vi "Word_Update_Table2.vi"(0 "report in":refnum<class "NI_report.lvclass">, 5 "start":cluster{"row":i32, "column":i32}, 9 "Table Ref":refnum<k7>, 11 "error in (no error)":errorcluster, 12 "value":string[][](array[string])) -> (4 "report out":refnum<class "NI_report.lvclass">, 15 "error out":errorcluster)   [LabVIEW 2020, in "NI_Word.lvclass"]
uses:
  <vilib>/Utility/NIReport.llb/Word/NI_Word.lvclass
  <vilib>/Utility/NIReport.llb/NI_report.lvclass
  C:/Program Files (x86)/National Instruments/LabVIEW 2020/vi.lib/Utility/NIReport.llb/NI_report.lvclass
  <vilib>/Utility/NIReport.llb/Word/NI_Word.lvclass/NI_Word.ctl
  <vilib>/Utility/NIReport.llb/NI_ReportGenerationCore.lvlib
panel:
  # "This is a copy of the Word_Update_Table.vi specifically used by\nthe MS Office Report Express VI to update the contents of\na table where the bookmark consists of a group of table cells."
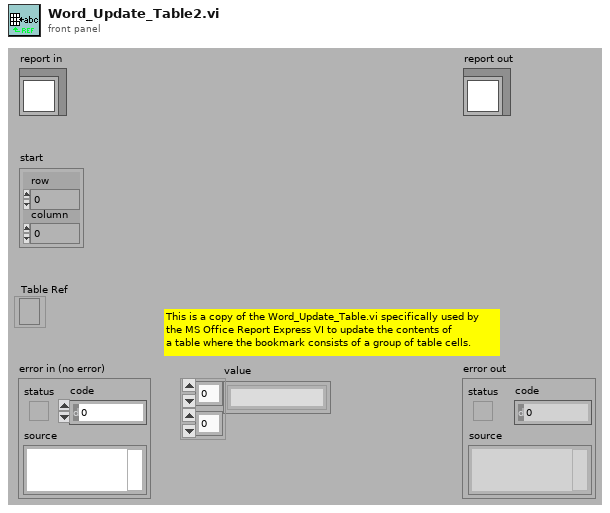
[diagram p1: front panel]
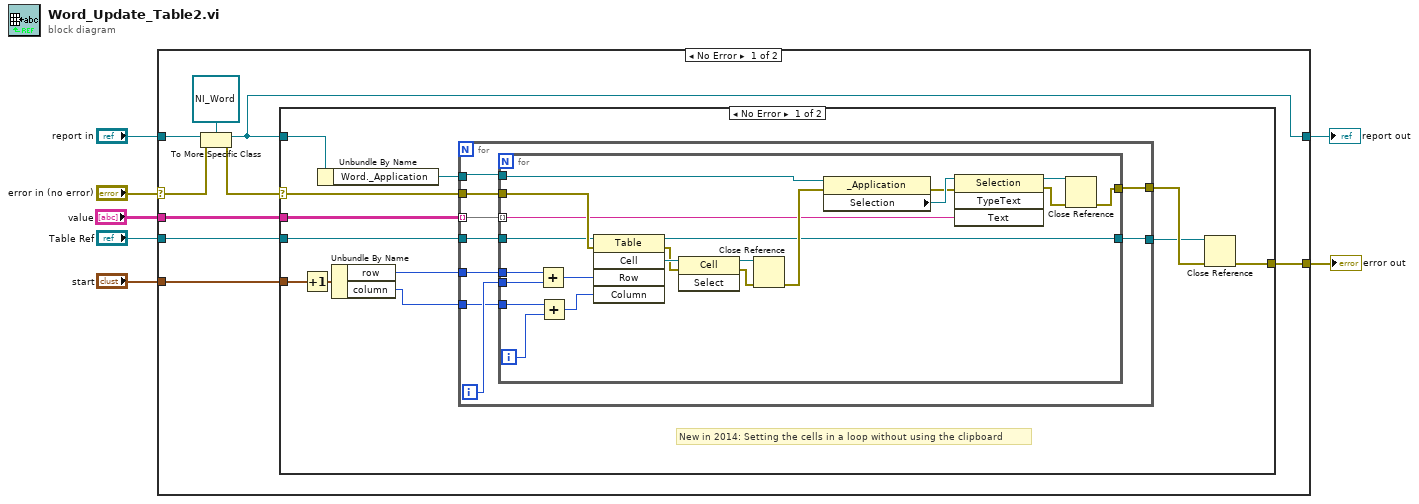
[diagram p0: block diagram]
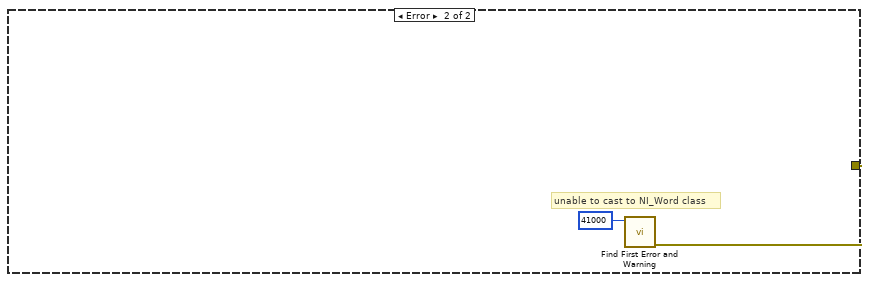
[diagram p2: hidden frame]
diagram:
  n1 = case shown="No Error" "error in (no error)" {
    selector: "error in (no error)" -> [w10 w62]
    tunnel: [w13 w62] -> w6
    tunnel: [w9 w61] -> w4
    tunnel: "report in" -> [w11 w61]
    tunnel: "value" -> [w16 _]
    tunnel: "start" -> [w15 _]
    tunnel: "Table Ref" -> [w14 _]
    frame No Error {
      n2 = To More Specific Class(target class=refnum<class "NI_Word.lvclass"> refnum ("report in"), reference=w11, error in=w10) -> (specific class reference=w9:refnum<class "NI_Word.lvclass">, error out=w8:errorcluster)
      n3 = case shown="No Error" w8 {
        selector: w8 -> [w23 _]
        tunnel: w16 -> [w24 _]
        tunnel: w15 -> [w27 _]
        tunnel: w14 -> [w21 _]
        tunnel: [w26 w59] -> w13
        tunnel: w9 -> [w25 _]
        frame No Error {
          # "New in 2014: Setting the cells in a loop without using the clipboard"
          n4 = Increment(x=w27) -> (x+1=w28:cluster{"row":i32, "column":i32})
          n5 = Unbundle By Name(w25) -> ("Word._Application"=w22:refnum<k7>)
          n6 = Unbundle By Name(w28) -> ("row"=w20:i32, "column"=w19:i32)
          n7 = for {
            tunnel: w24 -> [w37] mode=indexing
            tunnel: [w36] -> w17
            tunnel: [w35] -> w18
            tunnel: w23 -> [w33]
            tunnel: w22 -> [w32]
            tunnel: w21 -> [w31]
            tunnel: w20 -> [w30]
            tunnel: w19 -> [w29]
            i -> [w34]
            n8 = for {
              tunnel: w37 -> [w49] mode=indexing
              tunnel: [w53] -> w36
              tunnel: [w46] -> w35
              tunnel: w34 -> [w43]
              tunnel: w33 -> [w52]
              tunnel: w32 -> [w51]
              tunnel: w31 -> [w50]
              tunnel: w30 -> [w41]
              tunnel: w29 -> [w40]
              i -> [w42]
              n9 = Add(x=w41, y=w43) -> (x+y=w39:i32)
              n10 = Add(x=w40, y=w42) -> (x+y=w38:i32)
              n11 = invoke class="Table" method="Cell"(reference=w50, error in=w52, "Row"=w39, "Column"=w38) -> (reference out=w53:refnum<k7>, error out=w57:errorcluster, "Cell"=w58:refnum<k7>)  [unwired: 1 in, 2 out]
              n12 = invoke class="Cell" method="Select"(reference=w58, error in=w57) -> (reference out=w54:refnum<k7>, error out=w56:errorcluster)  [unwired: 1 in, 1 out]
              n13 = Close Reference(reference=w54, error in (no error)=w56) -> (error out=w55:errorcluster)
              n14 = property class="_Application"(reference=w51, error in=w55) -> (error out=w44:errorcluster, "Selection"=w45:refnum<k7>)  [unwired: 1 out]
              n15 = invoke class="Selection" method="TypeText"(reference=w45, error in=w44, "Text"=w49) -> (reference out=w47:refnum<k7>, error out=w48:errorcluster)  [unwired: 1 in, 2 out]
              n16 = Close Reference(reference=w47, error in (no error)=w48) -> (error out=w46:errorcluster)
            }
          }
          n17 = Close Reference(reference=w17, error in (no error)=w18) -> (error out=w26:errorcluster)
        }
        frame Error {
          # "unable to cast to NI_Word class"
          n18 = call <vilib>:"Find First Error and Warning.vi"("error code"=41000) -> ("error out"=w59:errorcluster)  [unwired: 2 in, 4 out]
        }
      }
    }
    frame Error {
    }
  }
  "error out" <- w6
  "report out" <- w4
